vi "Get Sensor Config Info.vi"(8 "error in":errorcluster, 11 "conn":u32) -> (0 "error out":errorcluster, 2 "Data":string[][](array[string]), 3 "PQresultStatus":T1(ring))   [LabVIEW 2018]
uses:
  PostgreSQL2LabVIEW/libpqlv/libpqlv.lvlib
  PostgreSQL2LabVIEW/libpqUtility/libpqutility.lvlib
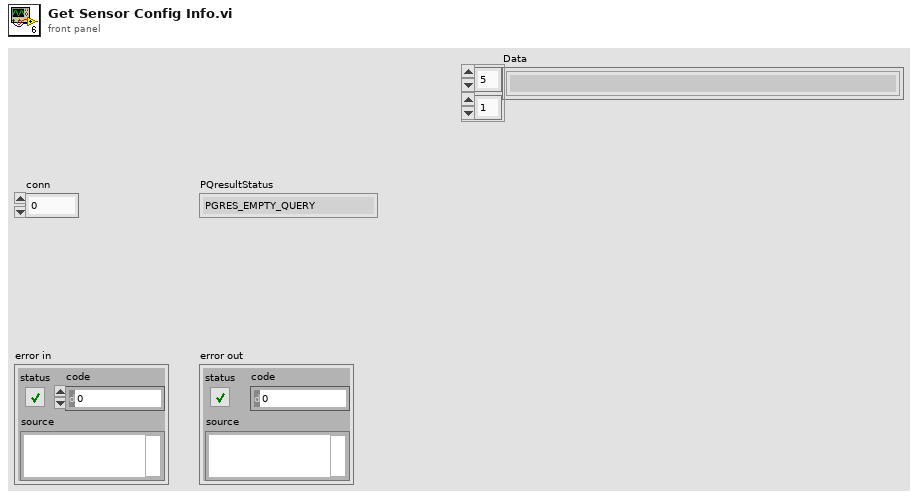
[diagram p1: front panel]
types:
  T1 = enum16{"PGRES_EMPTY_QUERY", "PGRES_COMMAND_OK", "PGRES_TUPLES_OK", "PGRES_COPY_OUT", "PGRES_COPY_IN", "PGRES_BAD_RESPONSE", "PGRES_NONFATAL_ERROR", "PGRES_FATAL_ERROR"}
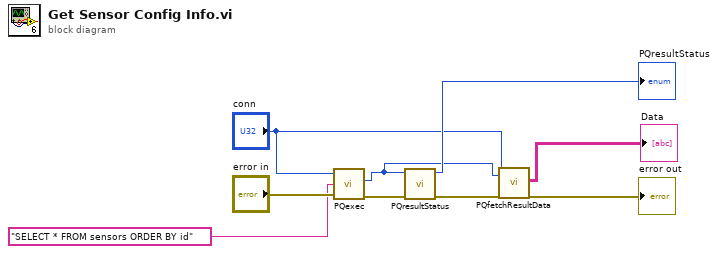
[diagram p0: block diagram]
diagram:
  n1 = call "PQexec.vi"("conn"="conn", "query"="SELECT * FROM sensors ORDER BY id" ("format string"), "error in (no error)"="error in") -> ("PGresult"=w5:u32, "error out"=w9:errorcluster)  [unwired: 2 in]
  n2 = call "PQresultStatus.vi"("error in (no error)"=w9, "res"=w5) -> ("error out"=w2:errorcluster, "PQresultStatus"=→"PQresultStatus":T1)  [unwired: 8 in]
  n3 = call "PQfetchResultData.vi"("conn"="conn", "res"=w5, "error in"=w2) -> ("Data"=→"Data":string[][], "error out"=→"error out":errorcluster)  [unwired: 11 in, 4 out]
